vi "LabVIEW - Convbox.vi"() -> ()   [LabVIEW 2019]
doc: "This simple example demonstrates <B>GPIB Read</B> and <B>GPIB Write</B>. A device connected to a GPIB bus can be written to or be read from using this VI. Enter the <B>GPIB Address</B> of the device, choose <B>Read from Instr</B>, <B>Write to Instr</B>, or <B>Write then Read</B>, type in the characters to be written, and run the VI. If you choose <B>Write then Read</B>, the VI will write to the device first, then read from the device. Before using this VI you should initialize the GPIB address according to the device's specifications with the \"GPIB Initialization\" function."
uses:
  <vilib>/dlg_ctls.llb/Space Constant.vi
  Status ConvBox.vi
  CheckListener ConvBox.vi
  <vilib>/Utility/error.llb/Clear Errors.vi
  <vilib>/Utility/error.llb/Error Cluster From Error Code.vi
panel:
  in  "GPIB Address":string="1"
  out "Characters Read":string
  in  "# Bytes to Read":i32=200
  in  "Characters to Write":string="*IDN?"
  in  "Operation":T1(ring)
  # "1. Enter the GPIB address of the device.\n2. Choose the operation to perform (read, write, or both). \n3. Enter a timeout value in milliseconds.\n4. Enter the number of bytes to read.\n5. Type in the characters to be written to the instrument.\n6. Run the VI. \n\nIf you choose the \"Write then Read\" operation, the VI will write to the device first, then read from the device.\nBefore using this VI, you should consider initializing the bus with the \"GPIB Initialization\" function."
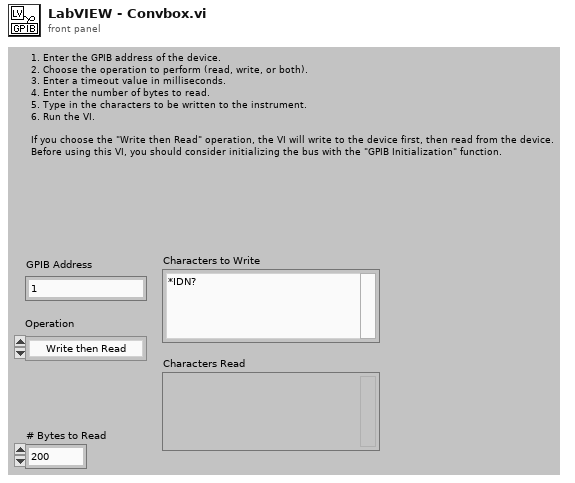
[diagram p1: front panel]
types:
  T1 = enum16{"Write then Read", "Write to Instr", "Read from Instr"}
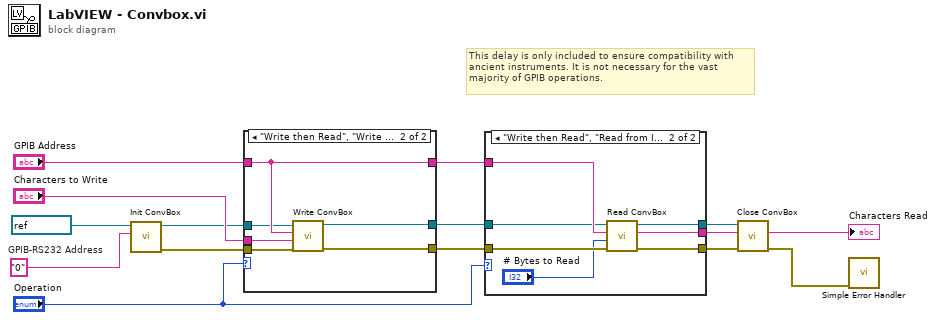
[diagram p0: block diagram]
diagram:
  w8 = "0"  # GPIB-RS232 Address
  # "This delay is only included to ensure compatibility with ancient instruments. It is not necessary for the vast majority of GPIB operations."
  n1 = call "Init ConvBox.vi"("Address"=w8, "Serial Port"=refnum<visa-resource-name> "Com1") -> ("error out"=w11:errorcluster, "Serial Port Out"=w10:refnum<visa-resource-name>)  [unwired: 8 in]
  n2 = case shown="\"Write then Read\", \"Write to Instr\"" "Operation" {
    tunnel: "GPIB Address" -> [w17 w23]
    tunnel: "Characters to Write" -> [_ w22]
    tunnel: [w17 w23] -> w4
    tunnel: [w15 w21] -> w2
    tunnel: w11 -> [w15 w20]
    tunnel: w10 -> [w16 w19]
    tunnel: [w16 w18] -> w3
    frame Default {
    }
    frame "Write then Read", "Write to Instr" {
      n3 = call "Write ConvBox.vi"("error in"=w20, "data"=w22, "address string"=w23, "VISA resource in"=w19) -> ("error out"=w21:errorcluster, "VISA resource out"=w18:refnum<visa-resource-name>)  [unwired: 5 in, 1 out]
    }
  }
  n4 = case shown="\"Write then Read\", \"Read from Instr\"" "Operation" {
    tunnel: w4 -> [_ w29]
    tunnel: [_ w30] -> w13
    tunnel: w2 -> [w25 w32]
    tunnel: [w25 w31] -> w7
    tunnel: w3 -> [w24 w27]
    tunnel: [w24 w26] -> w6
    frame Default {
    }
    frame "Write then Read", "Read from Instr" {
      n5 = call "Read ConvBox.vi"("error in"=w32, "byte count"="# Bytes to Read", "address string"=w29, "VISA resource in"=w27) -> ("error out"=w31:errorcluster, "data"=w30:string, "VISA resource out"=w26:refnum<visa-resource-name>)  [unwired: 4 in, 1 out]
    }
  }
  "Characters Read" <- w13
  n6 = call "Close ConvBox.vi"("error in (no error)"=w7, "Serial Port"=w6) -> ("error out"=w5:errorcluster)  [unwired: 9 in]
  n7 = call <vilib>:"Simple Error Handler.vi"("error in (no error)"=w5) -> ()  [unwired: 4 in, 5 out]
